vi "State_Machine.vi"(8 "error in (no error)":errorcluster caption="entrée d'erreur (pas d'erreur)", 11 "Delay en entrée":refnum<class "P2313_Scan_QRCode.lvclass">) -> (0 "error out":errorcluster caption="sortie d'erreur", 2 "Json_String":string, 3 "Delay en sortie":refnum<class "P2313_Scan_QRCode.lvclass">)   [LabVIEW 2020, in "Library Test.lvlib" / "P2313_Scan_QRCode.lvclass"]
uses:
  P2313_Scan_QRCode.lvclass
  C:/Users/ngarcin/OneDrive - Altyor/Standard TB/Suite TB45/Class/Test/Test (Default)/Test (Default).lvclass
  Popup/Class Popup Operator_Input Batch_AIS/Class Popup Operator_Input_PCRE.lvclass
  Commun VI/TypeDef/Variable Printable.ctl
  Popup/Class Popup (Main)/Class Popup (Main).lvclass
  JSON API/JSON Value/Set from JSON string.vi
  JSON API/JSON Value/JSON Value.lvclass
  JSON API/Variant JSON/Variant JSON.lvlib
  JSON API/Get Polymorphic/JSON GetSet.lvlib
  Commun VI/Library Commun.lvlib
  Test (Default)/Test (Default).lvclass
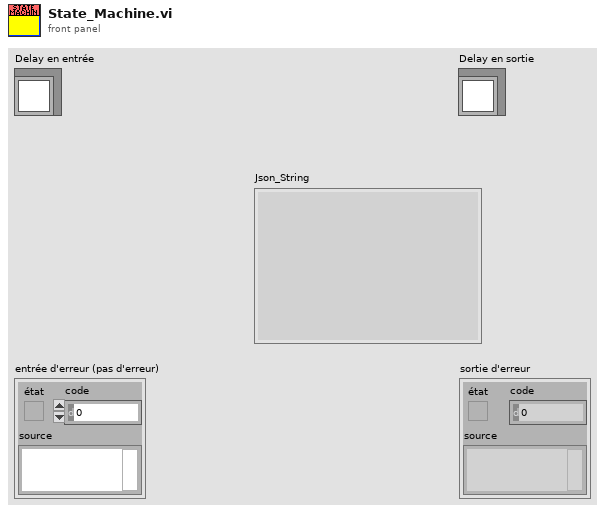
[diagram p1: front panel]
types:
  T1 = typedef "Variable Printable.ctl" = string
  T2 = enum16{"Get Variable", "Get All Variables", "Set Variable", "Delete Variable", "Delete All Variable"}
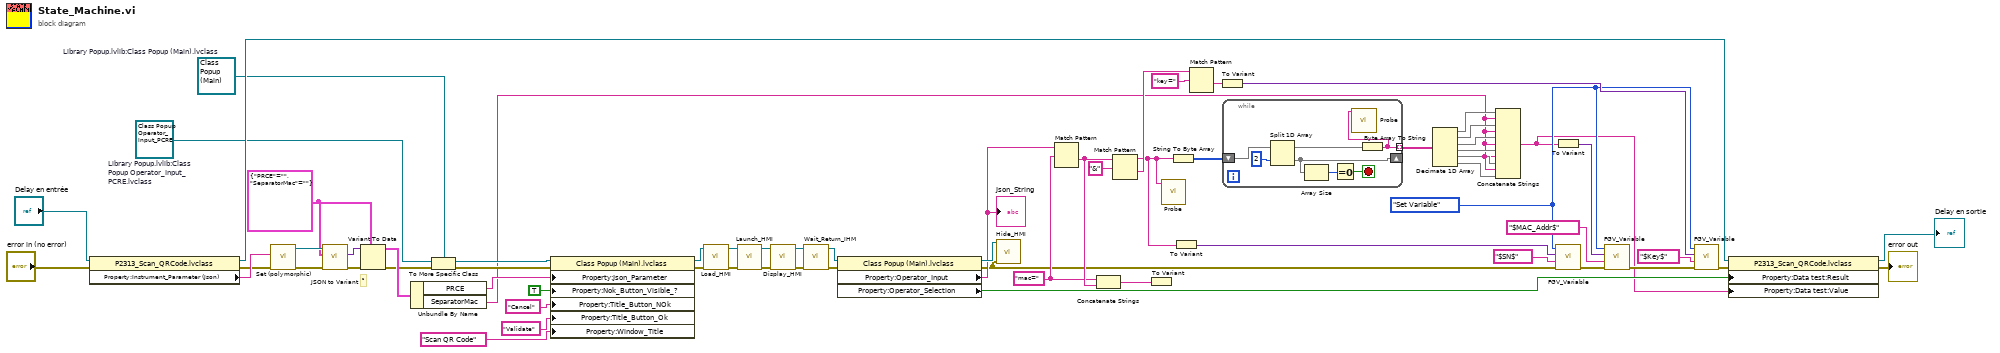
[diagram p0: block diagram]
diagram:
  w28 = refnum<class "Class Popup (Main).lvclass"> refnum  # Library Popup.lvlib:Class Popup (Main).lvclass
  w20 = "mac=" ("expression régulière")
  w5 = T2."Set Variable" ("Function")
  w40 = cluster{"PRCE":string, "SeparatorMac":string} {"PRCE"="", "SeparatorMac"=""}
  w27 = refnum<class "Class Popup Operator_Input_PCRE.lvclass"> refnum  # Library Popup.lvlib:Class Popup Operator_Input_PCRE.lvclass
  # "²"
  n1 = property class="P2313_Scan_QRCode.lvclass"(reference="Delay en entrée", error in="error in (no error)") -> (reference out=w46:refnum<class "P2313_Scan_QRCode.lvclass">, error out=w62:errorcluster, "Property:Instrument_Parameter (Json)"=w64:string)
  n2 = call-poly "Set (polymorphic).vi"("error in (no error)"=w62, "JSON stream"=w64) -> ("error out"=w42:errorcluster, "JSON Value out"=w44:refnum<class "JSON Value.lvclass">)  [unwired: 7 in, 1 out]
  n3 = call "JSON to Variant.vi"("error in (no error)"=w42, "Variant (Data Type)"=w40, "JSON Value"=w44) -> ("error out"=w43:errorcluster, "Variant out"=w41:variant)  [unwired: 7 in]
  n4 = Variant To Data(error in=w43, type=w40, Variant=w41) -> (data=w39:cluster{"PRCE":string, "SeparatorMac":string}, error out=w25:errorcluster)
  n5 = Unbundle By Name(w39) -> ("PRCE"=w38:string, "SeparatorMac"=w9:string)
  n6 = To More Specific Class(target class=w28, reference=w27, error in=w25) -> (specific class reference=w26:refnum<class "Class Popup (Main).lvclass">, error out=w24:errorcluster)
  n7 = property class="Class Popup (Main).lvclass"(reference=w26, error in=w24, "Property:Json_Parameter"=w38, "Property:Nok_Button_Visible_?"=TRUE ("Nok_Button_Visible_?"), "Property:Title_Button_NOk"="Cancel" ("Title_Button_NOk"), "Property:Title_Button_Ok"="Validate" ("Title_Button_Ok"), "Property:Window_Title"="Scan QR Code" ("Window_Title")) -> (reference out=w56:refnum<class "Class Popup (Main).lvclass">, error out=w55:errorcluster)
  n8 = call-dynamic "Load_HMI.vi"("error in (no error)"=w55, "Class Popup (Default) en entrée"=w56) -> ("error out"=w61:errorcluster, "Class Popup (Default) en sortie"=w60:refnum<class "Class Popup (Main).lvclass">)  [unwired: 8 in]
  n9 = call-dynamic "Launch_HMI.vi"("error in (no error)"=w61, "Class Popup (Default) en entrée"=w60) -> ("error out"=w59:errorcluster, "Class Popup (Default) en sortie"=w58:refnum<class "Class Popup (Main).lvclass">)  [unwired: 8 in]
  n10 = call-dynamic "Display_HMI.vi"("error in (no error)"=w59, "Class Popup (Default) en entrée"=w58) -> ("error out"=w22:errorcluster, "Class Popup (Default) en sortie"=w57:refnum<class "Class Popup (Main).lvclass">)  [unwired: 8 in]
  n11 = call-dynamic "Wait_Return_IHM.vi"("error in (no error)"=w22, "Class Popup (Default) en entrée"=w57) -> ("error out"=w23:errorcluster, "Class Popup (Default) en sortie"=w51:refnum<class "Class Popup (Main).lvclass">)  [unwired: 8 in]
  n12 = property class="Class Popup (Main).lvclass"(reference=w51, error in=w23) -> (reference out=w50:refnum<class "Class Popup (Main).lvclass">, error out=w8:errorcluster, "Property:Operator_Input"=w29:string, "Property:Operator_Selection"=w45:bool)
  "Json_String" <- w29
  n13 = call-dynamic "Hide_HMI.vi"("error in (no error)"=w8, "Class Popup (Default) en entrée"=w50) -> ()  [unwired: 8 in, 2 out]
  n14 = Match Pattern(string=w29, regular expression=w20) -> (after substring=w21:string)  [unwired: 1 in, 3 out]
  n15 = Concatenate Strings(w20, w21) -> (w19:string)
  n16 = Match Pattern(string=w21, regular expression="&" ("expression régulière")) -> (before substring=w1:string, after substring=w33:string)  [unwired: 1 in, 2 out]
  n17 = To Variant(anything=w19) -> ()  [unwired: 1 out]
  n18 = call "Probe.vi"("Message"=w1) -> ()  [unwired: 10 in, 1 out]
  n19 = String To Byte Array(string=w1) -> (unsigned byte array=w13:u8[])
  n20 = To Variant(anything=w1) -> (Variant=w6:variant)
  n21 = Match Pattern(string=w33, regular expression="key=" ("expression régulière")) -> (after substring=w31:string)  [unwired: 1 in, 3 out]
  n22 = To Variant(anything=w31) -> (Variant=w30:variant)
  n23 = while {
    tunnel: [w66] -> w12 mode=indexing
    shift-right: [w70] -> _
    shift-left: w13 -> [w72]
    stop <- w69 stop-if-true
    n24 = Split 1D Array(array=w72, index=2 ("indice")) -> (first subarray=w67:u8[], second subarray=w70:u8[])
    n25 = Array Size(array=w70) -> (size(s)=w68:i32)
    n26 = Equal To 0?(x=w68) -> (x = 0?=w69:bool)
    n27 = Byte Array To String(unsigned byte array=w67) -> (string=w66:string)
    n28 = call "Probe.vi"("Message"=w66) -> ()  [unwired: 10 in, 1 out]
  }
  n29 = Decimate 1D Array(w12) -> (w11:string[], w18:string[], w17:string[], w16:string[], w15:string[], w14:string[])
  n30 = Concatenate Strings(w11, w9, w18, w9, w17, w9, w16, w9, w15, w9, w14) -> (w2:string)
  n31 = To Variant(anything=w2) -> (Variant=w10:variant)
  n32 = call "FGV_Variable.vi"("error in (no error)"=w8, "Variable"=T1 "$SN$", "Data In"=w6, "Function"=w5) -> ("error out"=w7:errorcluster)  [unwired: 5 in, 2 out]
  n33 = call "FGV_Variable.vi"("error in (no error)"=w7, "Variable"=T1 "$MAC_Addr$", "Data In"=w10, "Function"=w5) -> ("error out"=w36:errorcluster)  [unwired: 5 in, 2 out]
  n34 = call "FGV_Variable.vi"("error in (no error)"=w36, "Variable"=T1 "$Key$" ("Variable Printable"), "Data In"=w30, "Function"=w5) -> ("error out"=w3:errorcluster)  [unwired: 5 in, 2 out]
  n35 = property class="P2313_Scan_QRCode.lvclass"(reference=w46, error in=w3, "Property:Data test:Result"=w45, "Property:Data test:Value"=w2) -> (reference out=→"Delay en sortie":refnum<class "P2313_Scan_QRCode.lvclass">, error out=→"error out":errorcluster)
